vi "UIRefs MFC Calibrated Gas.vi"(8 "error in (no error)":errorcluster, 11 "C100L in":refnum<class "C100L.lvclass">) -> (0 "error out":errorcluster, 3 "C100L out":refnum<class "C100L.lvclass">)   [LabVIEW 2021, in "C100L.lvlib" / "C100L.lvclass"]
uses:
  C100L.lvclass
  C100L.lvclass/C100L.ctl
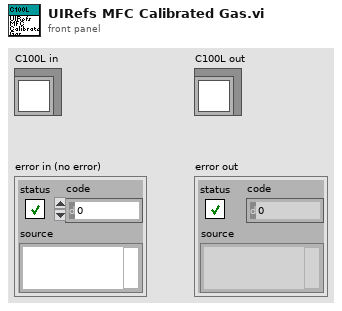
[diagram p1: front panel]
types:
  T1 = typedef "C100L.lvlib/C100L.lvclass/GCF Data.ctl" = map{string, dbl}
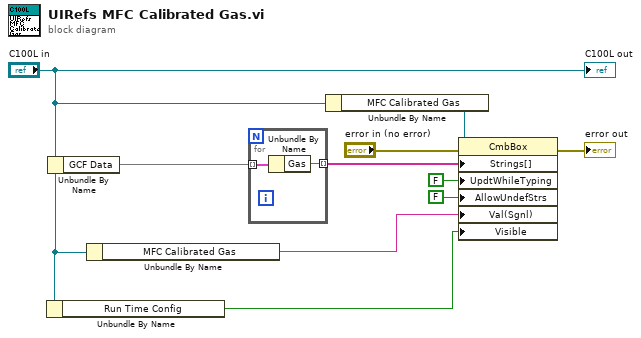
[diagram p0: block diagram]
diagram:
  n1 = Unbundle By Name("C100L in") -> ("Run Time Config"=w1:bool)
  n2 = Unbundle By Name("C100L in") -> ("GCF Data"=w9:T1)
  n3 = Unbundle By Name("C100L in") -> ("MFC Calibrated Gas"=w3:string)
  n4 = for {
    tunnel: [w11] -> w6 mode=indexing
    tunnel: w9 -> [w12] mode=indexing
    n5 = Unbundle By Name(w12) -> ("Gas"=w11:string)
  }
  n6 = Unbundle By Name("C100L in") -> ("MFC Calibrated Gas"=w10:refnum<vi>)
  n7 = property class="CmbBox"(reference=w10, error in="error in (no error)", "Strings[]"=w6, "UpdtWhileTyping"=FALSE ("Update While Typing?"), "AllowUndefStrs"=FALSE ("Allow Undefined Strings"), "Val(Sgnl)"=w3, "Visible"=w1) -> (error out=→"error out":errorcluster)  [unwired: 1 out]
  "C100L out" <- "C100L in"
